vi "CMD_SNAPSHOT.vi"(6 "Gantry in":refnum<class "Gantry.lvclass">, 8 "error in (no error)":errorcluster, 10 "Arguments":string[](array[string]), 11 "gScript Interpreter in":refnum<class "gScript Interpreter.lvclass">) -> (0 "error out":errorcluster, 3 "gScript Interpreter out":refnum<class "gScript Interpreter.lvclass">, 4 "Gantry out":refnum<class "Gantry.lvclass">)   [LabVIEW 2022 SP3, in "gScript Interpreter.lvclass"]
uses:
  gScript Interpreter.lvclass
  Shared Components/Gantry Class/Gantry.lvclass
  Shared Components/FlexWorktable/FlexWorktable.lvclass
panel:
  in  "Continue":bool
  out "Preview":T1(plugin-control)
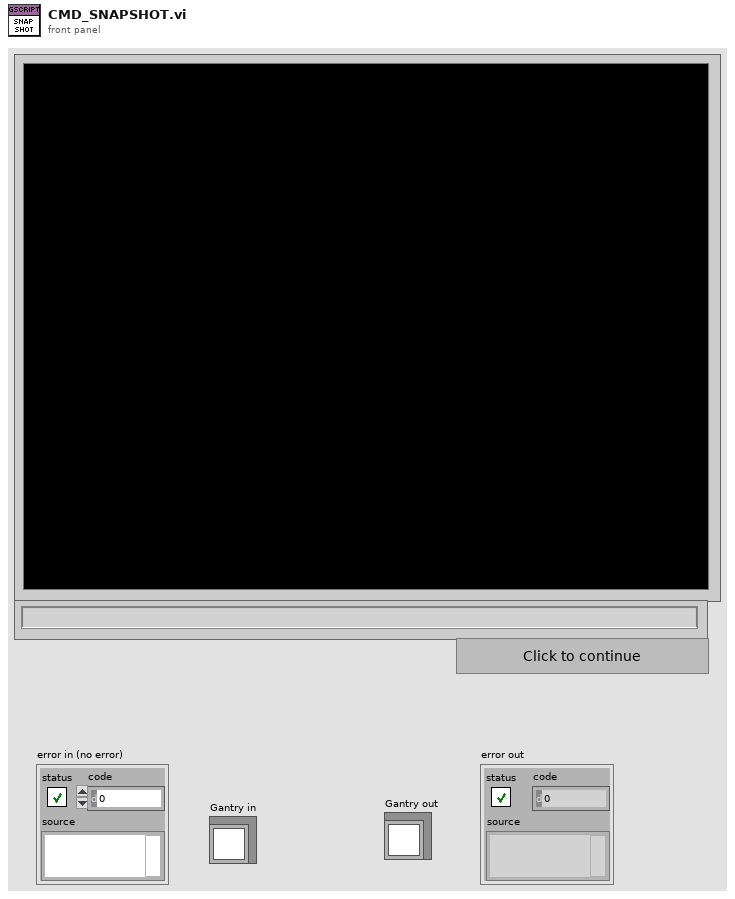
[diagram p1: front panel]
types:
  T1 = typedef "IMAQ Image.ctl" = refnum<image>
  T2 = typedef "Image Type" = u32
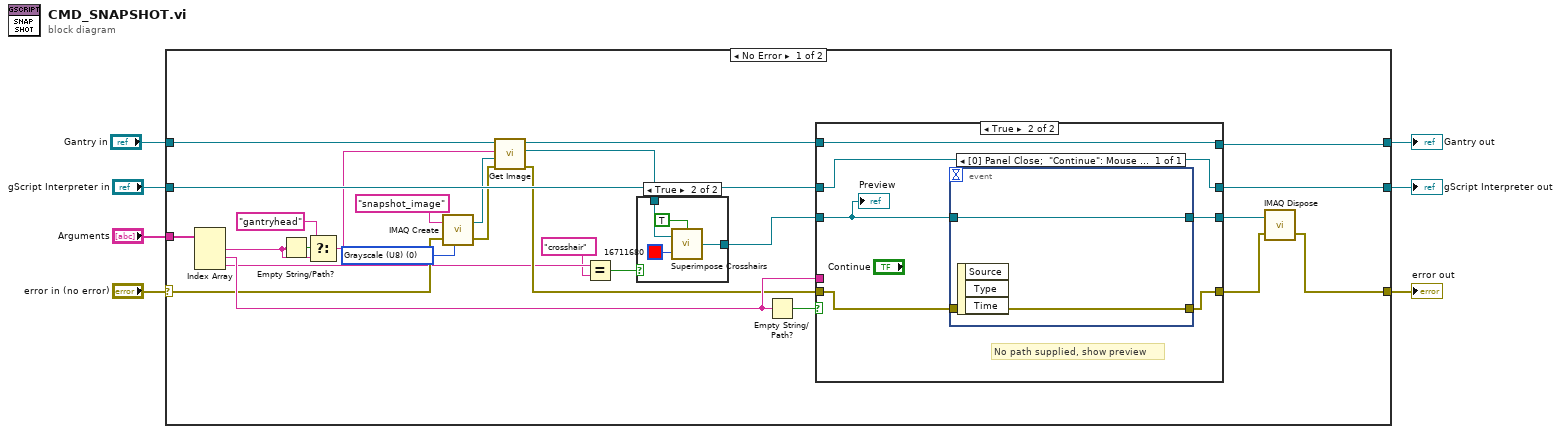
[diagram p0: block diagram]
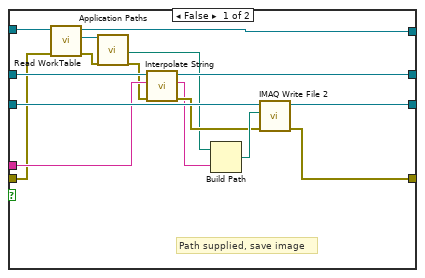
[diagram p3: hidden frame]
diagram:
  n1 = case shown="No Error" "error in (no error)" {
    selector: "error in (no error)" -> [w26 w65]
    tunnel: [w30 w65] -> w6
    tunnel: [w27 w64] -> w4
    tunnel: "gScript Interpreter in" -> [w28 w64]
    tunnel: "Arguments" -> [w33 _]
    tunnel: "Gantry in" -> [w32 w63]
    tunnel: [w31 w63] -> w1
    frame No Error {
      w8 = T2 0 items=["Grayscale (U8)", "Grayscale (I16)", "Grayscale (SGL)", "Complex (CSG)", "RGB (U32)", "HSL (U32)", "RGB (U64)", "Grayscale (U16)"] ("Image Type")
      n2 = Index Array(array=w33) -> (element #1=w16:string, element #2=w29:string, element #3=w13:string)  [unwired: 3 in]
      n3 = Empty String/Path?(string/path=w16) -> (empty?=w17:bool)
      n4 = Select(t="gantryhead", s=w17, f=w16) -> (s? t:f=w15:string)
      n5 = call "IMAQ Create"("Image Name"="snapshot_image", "Image Type"=w8, "error in (no error)"=w26) -> ("New Image"=w24:T1, "error out"=w23:errorcluster)  [unwired: 2 in]
      n6 = call-dynamic "Get Image.vi"("error in"=w23, "Image In"=w24, "Camera Name"=w15, "Gantry in"=w32) -> ("error out"=w20:errorcluster, "Image Out"=w12:T1, "Gantry out"=w22:refnum<class "Gantry.lvclass">)  [unwired: 4 in, 1 out]
      n7 = Equal?(x=w13, y="crosshair") -> (x = y?=w10:bool)
      n8 = case shown="True" w10 {
        tunnel: w12 -> [w34 w38]
        tunnel: [w34 w37] -> w11
        frame False {
        }
        frame True {
          n9 = call "Superimpose Crosshairs.vi"("Merge into Image"=TRUE, "Grid Line Color"=u32 16711680, "Refnum in"=w38) -> ("Refnum out"=w37:T1)
        }
      }
      n10 = Empty String/Path?(string/path=w29) -> (empty?=w21:bool)
      n11 = case shown="True" w21 {
        tunnel: w22 -> [w45 w60]
        tunnel: w20 -> [w43 w59]
        tunnel: w11 -> [w54 w57]
        tunnel: w29 -> [w47 _]
        tunnel: [w44 w60] -> w31
        tunnel: [w52 w56] -> w19
        tunnel: [w51 w58] -> w18
        tunnel: w28 -> [w50 w55]
        tunnel: [w48 w55] -> w27
        frame False {
          # "Path supplied, save image"
          n12 = call-dynamic "Read WorkTable.vi"("error in"=w43, "Gantry Class in"=w45) -> ("error out"=w41:errorcluster, "Worktable"=w42:refnum<class "FlexWorktable.lvclass">, "Gantry Class out"=w44:refnum<class "Gantry.lvclass">)  [unwired: 7 in]
          n13 = call "Application Paths.vi"("FlexWorktable in"=w42, "error in (no error)"=w41) -> ("Logs Path"=w39:path, "error out"=w40:errorcluster)  [unwired: 11 in, 5 out]
          n14 = call-dynamic "Interpolate String.vi"("error in (no error)"=w40, "Input String"=w47, "gScript Interpreter in"=w50) -> ("error out"=w49:errorcluster, "Output String"=w46:string, "gScript Interpreter out"=w48:refnum<class "gScript Interpreter.lvclass">)  [unwired: 6 in]
          n15 = Build Path(base path=w39, name or relative path=w46) -> (appended path=w53:path)
          n16 = call-poly "IMAQ Write File 2"("error in (no error)"=w49, "File Path"=w53, "Image"=w54) -> ("error out"=w51:errorcluster, "Image Out (duplicate)"=w52:T1)  [unwired: 7 in]
        }
        frame True {
          # "No path supplied, show preview"
          n17 = event shown="[0] Panel Close;  \"Continue\": Mouse Up;  Key Down" {
            selector: _ -> [_]
            dyn-events: _ -> [_]
            timeout: _ -> [_]
            tunnel: w59 -> [w62]
            tunnel: [w62] -> w58
            tunnel: w57 -> [w61]
            tunnel: [w61] -> w56
            event Panel Close; "Continue": Mouse Up; Key Down {
              n18 = event-data() -> ()  [unwired: 1 in, 3 out]
            }
          }
          "Preview" <- w57
        }
      }
      n19 = call "IMAQ Dispose"("Image"=w19, "error in (no error)"=w18) -> ("error out"=w30:errorcluster)  [unwired: 4 in]
    }
    frame Error {
    }
  }
  "error out" <- w6
  "gScript Interpreter out" <- w4
  "Gantry out" <- w1
